vi "TAT_Varient Creater.vi"(8 "error in (no error)":errorcluster) -> (0 "error out":errorcluster)   [LabVIEW 2017]
uses:
  <vilib>/Utility/config.llb/Read Key (I32).vi
  <vilib>/Utility/config.llb/Read Key (String).vi
  <vilib>/Utility/config.llb/Write Key (U32).vi
  <vilib>/Utility/config.llb/Write Key (String).vi
  <vilib>/Utility/config.llb/NI_LVConfig.lvlib
panel:
  in  "TORISHI CODE":string
  in  "PART NUMBER":string
  in  "Delete Square":bool
  in  "EDIT & SAVE":bool
  in  "Varient Details":string[][](table)
  in  "BATCH SIZE":u16=1 min=1 max=100 step=1
  in  "VARIENT NUMBER":u16=1 min=1 max=100 step=1
  in  "HOME":bool
  in  "UPDATE TABLE":bool
  in  "PART NAME":string(combo)
  # "Varient Creater"
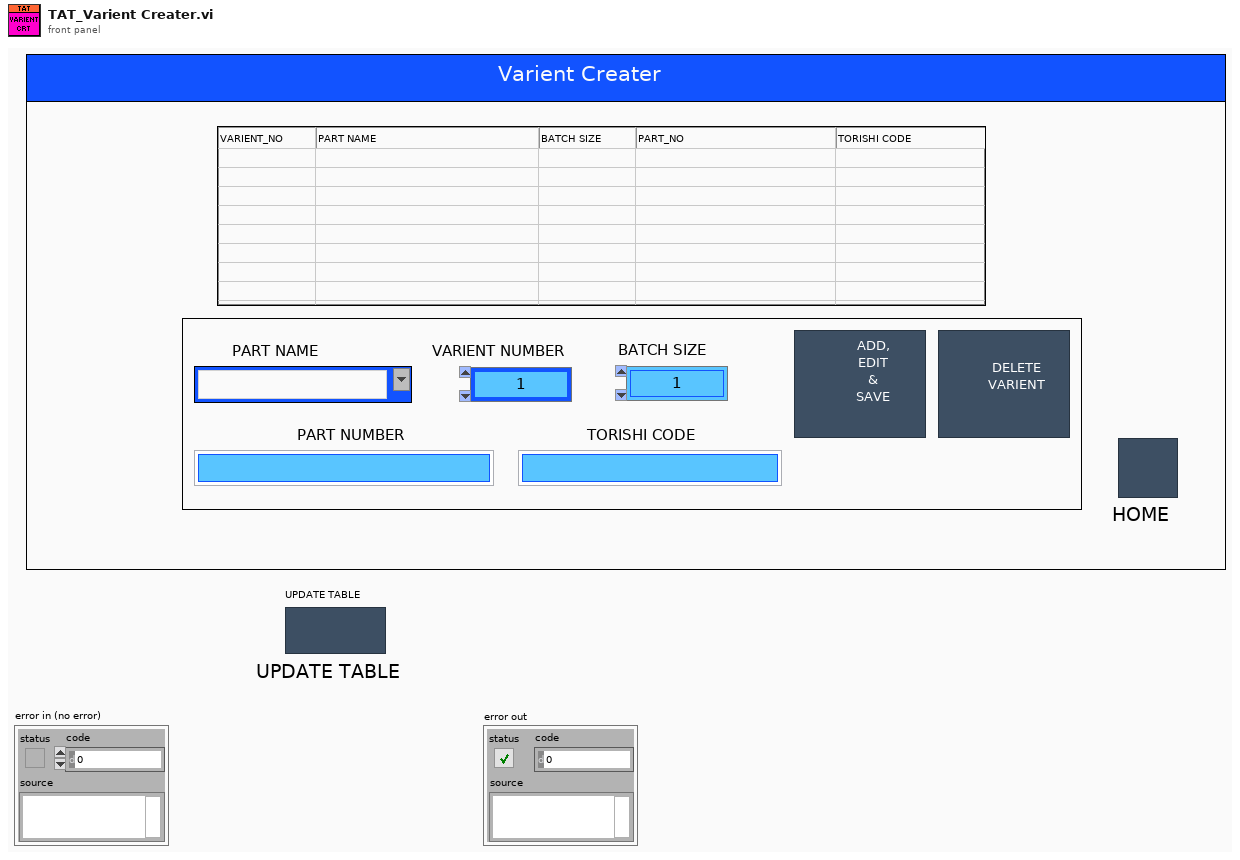
[diagram p1: front panel]
types:
  T1 = enum32{"invalid app kind", "Development System", "Run Time System", "Student Edition", "Embedded LabVIEW", "Evaluation", "Custom"}
  T2 = typedef "NI_LVConfig.lvlib/Config Data RefNum.ctl" = refnum<k1>
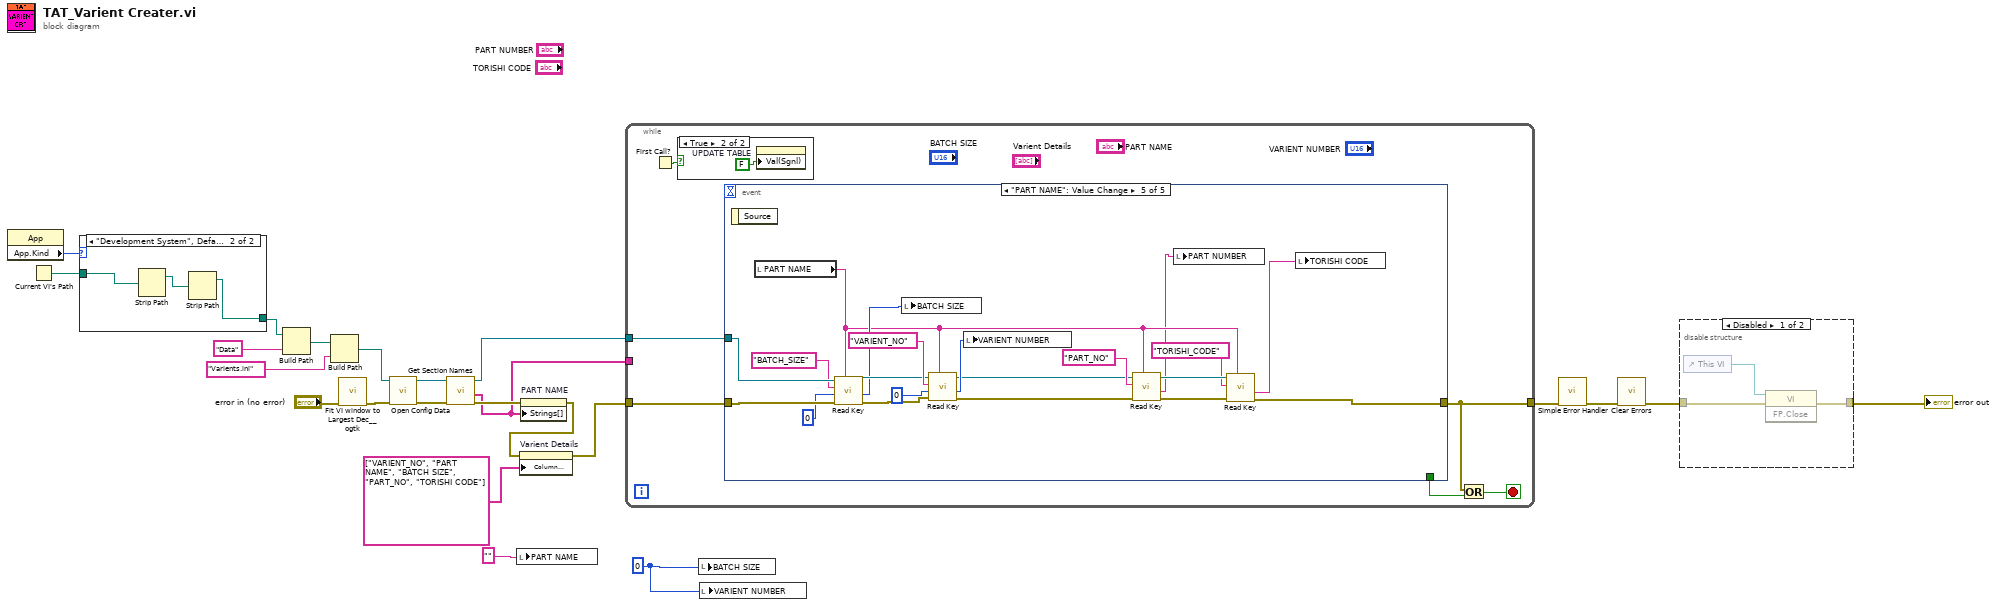
[diagram p0: block diagram]
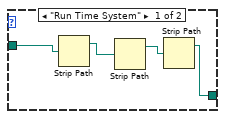
[diagram p3: hidden frame]
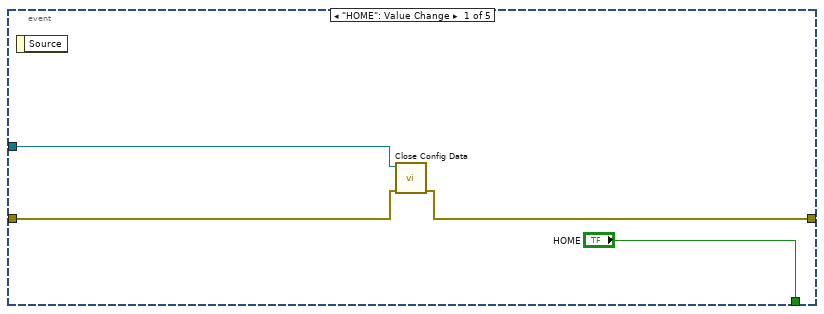
[diagram p5: hidden frame]
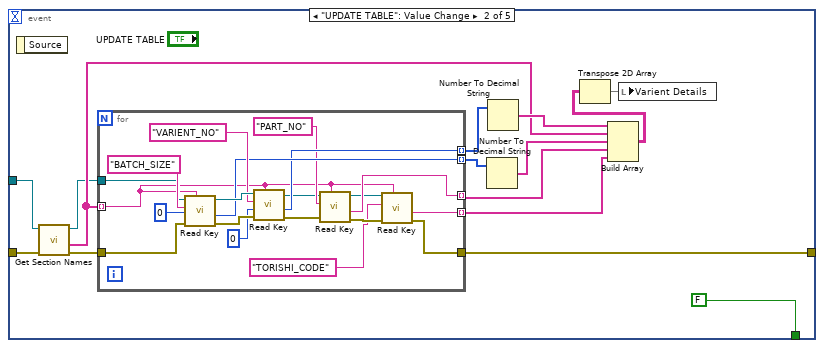
[diagram p6: hidden frame]
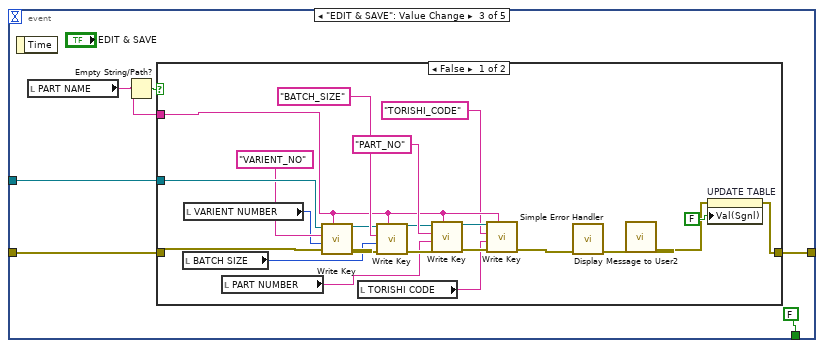
[diagram p7: hidden frame]
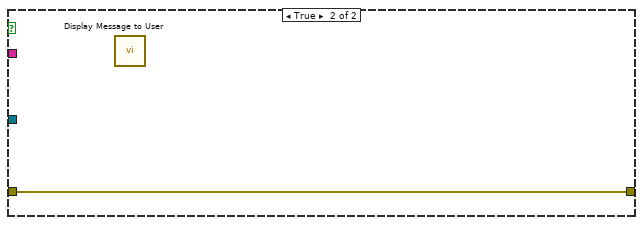
[diagram p8: hidden frame]
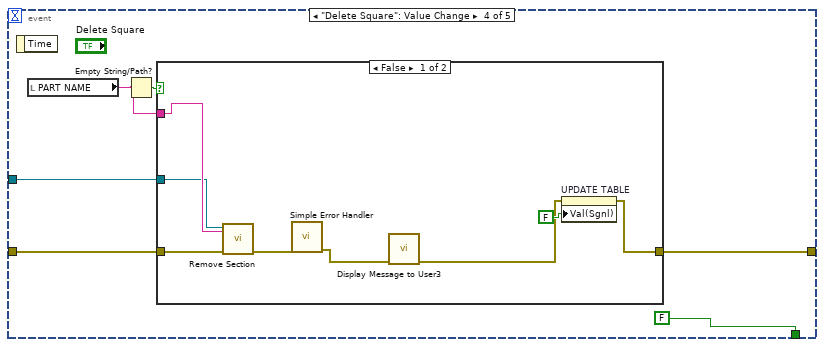
[diagram p9: hidden frame]
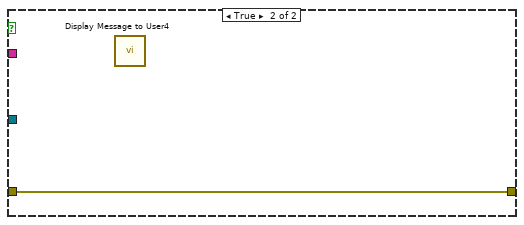
[diagram p10: hidden frame]
diagram:
  w1 = 0 ("default value")
  n1 = property class="App"() -> ("App.Kind"=w18:T1)  [unwired: 2 in, 2 out]
  n2 = Current VI's Path() -> (path=w19:path)
  n3 = case shown="\"Development System\", Default" w18 {
    tunnel: w19 -> [w25 w29]
    tunnel: [w24 w28] -> w16
    frame "Run Time System" {
      n4 = Strip Path(path=w25) -> (stripped path=w27:path)  [unwired: 1 out]
      n5 = Strip Path(path=w27) -> (stripped path=w26:path)  [unwired: 1 out]
      n6 = Strip Path(path=w26) -> (stripped path=w24:path)  [unwired: 1 out]
    }
    frame "Development System", Default {
      n7 = Strip Path(path=w29) -> (stripped path=w30:path)  [unwired: 1 out]
      n8 = Strip Path(path=w30) -> (stripped path=w28:path)  [unwired: 1 out]
    }
  }
  n9 = Build Path(base path=w16, name or relative path="Data") -> (appended path=w17:path)
  n10 = Build Path(base path=w17, name or relative path="Varients.ini") -> (appended path=w15:path)
  n11 = call <userlib>:"Fit VI window to Largest Dec__ogtk.vi"("error in (no error)"="error in (no error)") -> ("error out"=w9:errorcluster)  [unwired: 5 in, 1 out]
  n12 = call <vilib>:"Open Config Data.vi"("error in (no error)"=w9, "configuration file path"=w15) -> ("error out"=w11:errorcluster, "refnum"=w12:T2)  [unwired: 7 in, 1 out]
  n13 = call <vilib>:"Get Section Names.vi"("error in (no error)"=w11, "refnum"=w12) -> ("error out"=w10:errorcluster, "section names"=w3:string[], "refnum out"=w7:T2)  [unwired: 7 in]
  n14 = local write "PART NAME"("" ("name or relative path")) -> ()
  n15 = property on="PART NAME" class="CmbBox"(error in=w10, "Strings[]"=w3) -> (error out=w6:errorcluster)  [unwired: 1 in, 1 out]
  n16 = property on="Varient Details" class="Tbl (strict)"(error in=w6, "Column Headers[]"=string[] ["VARIENT_NO", "PART NAME", "BATCH SIZE", "PART_NO", "TORISHI CODE"] ("Column Header Strings[]")) -> (error out=w5:errorcluster)  [unwired: 1 in, 1 out]
  n17 = while {
    tunnel: w5 -> [w35]
    tunnel: [w33] -> w20
    tunnel: w7 -> [w32]
    tunnel: w3 -> [_]
    stop <- w34 stop-if-true
    n18 = First Call?() -> (First Call?: T/F=w31:bool)
    n19 = case shown="True" w31 {
      frame False {
      }
      frame True {
        n20 = property on="UPDATE TABLE" class="Bool (strict)"("Val(Sgnl)"=FALSE) -> ()  [unwired: 2 in, 2 out]
      }
    }
    n21 = event shown="[4] \"PART NAME\": Value Change" {
      selector: _ -> [_ _ _ _ _]
      dyn-events: _ -> [_ _ _ _ _]
      timeout: _ -> [_ _ _ _ _]
      tunnel: ["HOME" FALSE ("stop") FALSE ("stop") FALSE ("stop") _] -> w36
      tunnel: w35 -> [w40 w48 w78 w107 w140]
      tunnel: [w39 w55 w81 w110 w127] -> w33
      tunnel: w32 -> [w38 w45 w79 w108 w139]
      event "HOME": Value Change {
        n22 = event-data() -> ()  [unwired: 1 in, 1 out]
        n23 = call <vilib>:"Close Config Data.vi"("error in (no error)"=w40, "refnum"=w38) -> ("error out"=w39:errorcluster)  [unwired: 8 in, 1 out]
      }
      event "UPDATE TABLE": Value Change {
        n24 = event-data() -> ()  [unwired: 1 in, 1 out]
        n25 = call <vilib>:"Get Section Names.vi"("error in (no error)"=w48, "refnum"=w45) -> ("error out"=w47:errorcluster, "section names"=w46:string[], "refnum out"=w44:T2)  [unwired: 7 in]
        n26 = for {
          tunnel: [w61] -> w55
          tunnel: w47 -> [w70]
          tunnel: w46 -> [w58] mode=indexing
          tunnel: w44 -> [w69]
          tunnel: [w68] -> w53 mode=indexing
          tunnel: [w67] -> w54 mode=indexing
          tunnel: [w63] -> w43 mode=indexing
          tunnel: [w57] -> w42 mode=indexing
          n27 = call-poly <vilib>:"Read Key.vi"("section"=w58, "error in (no error)"=w70, "default value"=0, "key"="BATCH_SIZE", "refnum"=w69) -> ("error out"=w76:errorcluster, "value"=w68:i32, "refnum out"=w75:T2)  [unwired: 3 in, 1 out]
          n28 = call-poly <vilib>:"Read Key.vi"("section"=w58, "error in (no error)"=w76, "default value"=0, "key"="VARIENT_NO", "refnum"=w75) -> ("error out"=w66:errorcluster, "value"=w67:i32, "refnum out"=w64:T2)  [unwired: 3 in, 1 out]
          n29 = call-poly <vilib>:"Read Key.vi"("section"=w58, "error in (no error)"=w66, "key"="PART_NO", "refnum"=w64) -> ("error out"=w62:errorcluster, "value"=w63:string, "refnum out"=w60:T2)  [unwired: 4 in, 1 out]
          n30 = call-poly <vilib>:"Read Key.vi"("section"=w58, "error in (no error)"=w62, "key"="TORISHI_CODE", "refnum"=w60) -> ("error out"=w61:errorcluster, "value"=w57:string)  [unwired: 4 in, 2 out]
        }
        n31 = Number To Decimal String(number=w53) -> (decimal integer string=w52:string[])  [unwired: 1 in]
        n32 = Number To Decimal String(number=w54) -> (decimal integer string=w49:string[])  [unwired: 1 in]
        n33 = Build Array(w49, w46, w52, w43, w42) -> (w51:string[][])
        n34 = Transpose 2D Array(2D array=w51) -> (transposed array=w50:string[][])
        n35 = local write "Varient Details"(w50) -> ()
      }
      event "EDIT & SAVE": Value Change {
        n36 = event-data() -> ()  [unwired: 1 in, 1 out]
        n37 = local read "PART NAME"() -> (w77:string)
        n38 = Empty String/Path?(string/path=w77) -> (empty?=w80:bool)
        n39 = case shown="False" w80 {
          tunnel: w78 -> [w103 w105]
          tunnel: [w97 w105] -> w81
          tunnel: w79 -> [w101 _]
          tunnel: w77 -> [w86 _]
          frame False {
            n40 = local read "BATCH SIZE"() -> (w96:u16)
            n41 = local read "VARIENT NUMBER"() -> (w95:u16)
            n42 = local read "PART NUMBER"() -> (w83:string)
            n43 = call-poly <vilib>:"Write Key.vi"("section"=w86, "error in (no error)"=w103, "value"=w95, "key"="VARIENT_NO", "refnum"=w101) -> ("error out"=w102:errorcluster, "refnum out"=w100:T2)  [unwired: 4 in, 1 out]
            n44 = local read "TORISHI CODE"() -> (w84:string)
            n45 = call-poly <vilib>:"Write Key.vi"("section"=w86, "error in (no error)"=w102, "value"=w96, "key"="BATCH_SIZE", "refnum"=w100) -> ("error out"=w90:errorcluster, "refnum out"=w87:T2)  [unwired: 4 in, 1 out]
            n46 = call-poly <vilib>:"Write Key.vi"("section"=w86, "error in (no error)"=w90, "value"=w83, "key"="PART_NO", "refnum"=w87) -> ("error out"=w91:errorcluster, "refnum out"=w92:T2)  [unwired: 4 in, 1 out]
            n47 = call-poly <vilib>:"Write Key.vi"("section"=w86, "error in (no error)"=w91, "value"=w84, "key"="TORISHI_CODE", "refnum"=w92) -> ("error out"=w89:errorcluster)  [unwired: 4 in, 2 out]
            n48 = call <vilib>:"Simple Error Handler.vi"("error in (no error)"=w89) -> ("error out"=w94:errorcluster)  [unwired: 4 in, 4 out]
            n49 = call "Display Message to User2"("error in (no error)"=w94) -> ("error out"=w93:errorcluster)  [unwired: 9 in, 1 out]
            n50 = property on="UPDATE TABLE" class="Bool (strict)"(error in=w93, "Val(Sgnl)"=FALSE) -> (error out=w97:errorcluster)  [unwired: 1 in, 1 out]
          }
          frame True {
            n51 = call "Display Message to User"() -> ()  [unwired: 10 in, 2 out]
          }
        }
      }
      event "Delete Square": Value Change {
        n52 = event-data() -> ()  [unwired: 1 in, 1 out]
        n53 = local read "PART NAME"() -> (w106:string)
        n54 = Empty String/Path?(string/path=w106) -> (empty?=w109:bool)
        n55 = case shown="False" w109 {
          tunnel: w107 -> [w113 w120]
          tunnel: [w118 w120] -> w110
          tunnel: w108 -> [w114 _]
          tunnel: w106 -> [w115 _]
          frame False {
            n56 = call <vilib>:"Remove Section.vi"("section"=w115, "error in (no error)"=w113, "refnum"=w114) -> ("error out"=w112:errorcluster)  [unwired: 6 in, 2 out]
            n57 = call <vilib>:"Simple Error Handler.vi"("error in (no error)"=w112) -> ("error out"=w117:errorcluster)  [unwired: 4 in, 4 out]
            n58 = call "Display Message to User3"("error in (no error)"=w117) -> ("error out"=w116:errorcluster)  [unwired: 9 in, 1 out]
            n59 = property on="UPDATE TABLE" class="Bool (strict)"(error in=w116, "Val(Sgnl)"=FALSE) -> (error out=w118:errorcluster)  [unwired: 1 in, 1 out]
          }
          frame True {
            n60 = call "Display Message to User4"() -> ()  [unwired: 10 in, 2 out]
          }
        }
      }
      event "PART NAME": Value Change {
        n61 = event-data() -> ()  [unwired: 1 in, 1 out]
        n62 = local read "PART NAME"() -> (w123:string)
        n63 = call-poly <vilib>:"Read Key.vi"("section"=w123, "error in (no error)"=w140, "default value"=0, "key"="BATCH_SIZE", "refnum"=w139) -> ("error out"=w136:errorcluster, "value"=w131:i32, "refnum out"=w135:T2)  [unwired: 3 in, 1 out]
        n64 = local write "BATCH SIZE"(w131) -> ()
        n65 = call-poly <vilib>:"Read Key.vi"("section"=w123, "error in (no error)"=w136, "default value"=0, "key"="VARIENT_NO", "refnum"=w135) -> ("error out"=w128:errorcluster, "value"=w134:i32, "refnum out"=w124:T2)  [unwired: 3 in, 1 out]
        n66 = local write "VARIENT NUMBER"(w134) -> ()
        n67 = call-poly <vilib>:"Read Key.vi"("section"=w123, "error in (no error)"=w128, "key"="PART_NO", "refnum"=w124) -> ("error out"=w129:errorcluster, "value"=w122:string, "refnum out"=w130:T2)  [unwired: 4 in, 1 out]
        n68 = local write "PART NUMBER"(w122) -> ()
        n69 = call-poly <vilib>:"Read Key.vi"("section"=w123, "error in (no error)"=w129, "key"="TORISHI_CODE", "refnum"=w130) -> ("error out"=w127:errorcluster, "value"=w121:string)  [unwired: 4 in, 2 out]
        n70 = local write "TORISHI CODE"(w121) -> ()
      }
    }
    n71 = Or(x=w33, y=w36) -> (x .or. y?=w34:bool)
  }
  n72 = local write "BATCH SIZE"(w1) -> ()
  n73 = local write "VARIENT NUMBER"(w1) -> ()
  n74 = call <vilib>:"Simple Error Handler.vi"("error in (no error)"=w20) -> ("error out"=w23:errorcluster)  [unwired: 4 in, 4 out]
  n75 = call <vilib>:"Clear Errors.vi"("error in (no error)"=w23) -> ("error out"=w22:errorcluster)  [unwired: 5 in, 1 out]
  n76 = disable-structure shown="Disabled" {
    disable-tunnel: w22 -> [w143 w144]
    disable-tunnel: [w142 w144] -> w21
    frame Disabled {
      n77 = control-ref of="This VI"() -> (w141:refnum<vi>)
      n78 = invoke class="VI" method="FP.Close"(reference=w141, error in=w143) -> (error out=w142:errorcluster)  [unwired: 1 in, 2 out]
    }
    frame Enabled {
    }
  }
  "error out" <- w21
